vi "AlliGator Correct Dead Left Columns.vi"(8 "error in (no error)":errorcluster, 11 "Image Pixels":sgl[][](array[numeric])) -> (0 "error out":errorcluster, 3 "Corrected Image Pixels":sgl[][](array[numeric]))   [LabVIEW 2021, in "AlliGator Files.lvlib"]
doc: "Corrects for 1-every-other dead columns in the left half of a SPAD512S detector."
uses:
  AlliGator Files.lvlib
  35e40605-0482-421d-9502-94a1263c656b.vi
  <vilib>/Analysis/Matrix/Numeric/Conversions/Array To Matrix - RA2.vi
  <vilib>/Analysis/Matrix/Numeric/Conversions/Matrix To Array - RM.vi
  <vilib>/Analysis/Matrix/NI_Matrix.lvlib
panel:
  # "see the AlliGator License on the block diagram (Ctrl+E or Window:Show Block Diagram)"
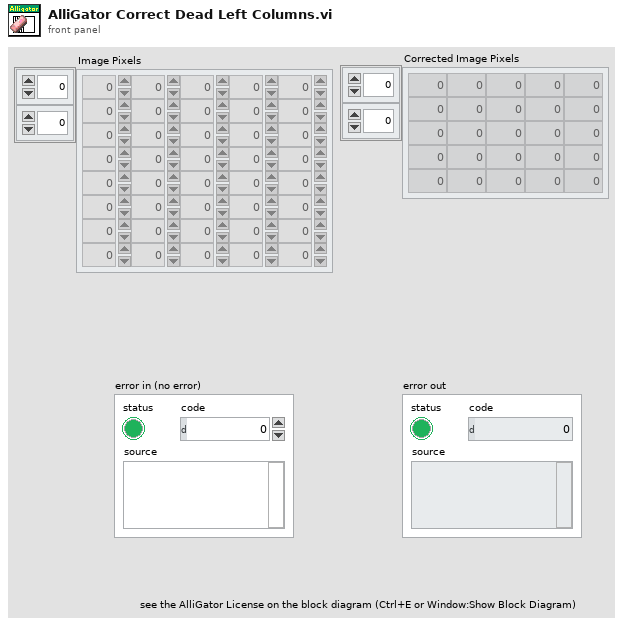
[diagram p1: front panel]
types:
  T1 = typedef "NI_Matrix.lvlib/RealMatrix.ctl" = dbl[][]
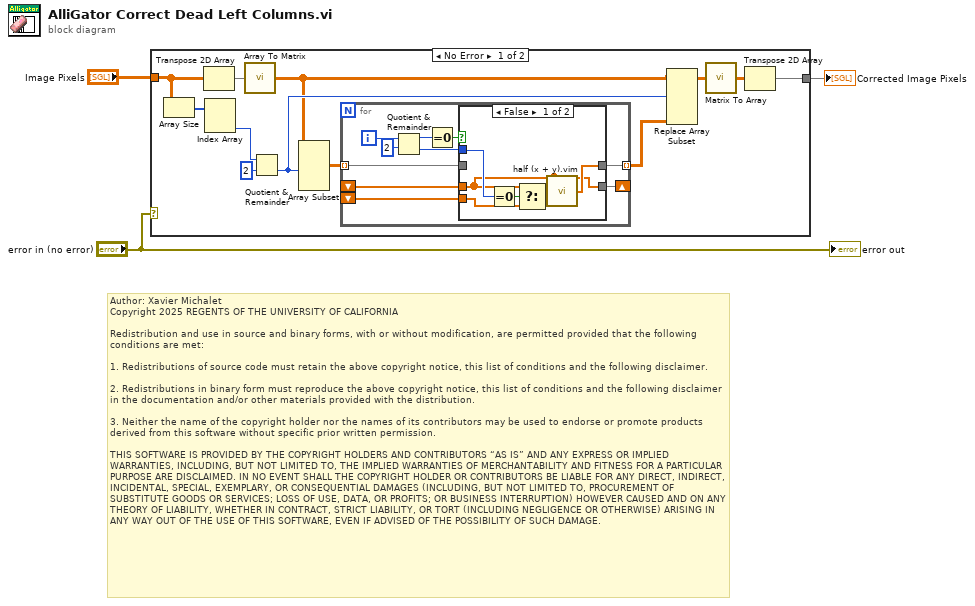
[diagram p0: block diagram]
diagram:
  # "Author: Xavier Michalet\nCopyright 2025 REGENTS OF THE UNIVERSITY OF CALIFORNIA\n\nRedistribution and use in source and binary forms, with or without modification, are permitted provided that the following conditions are met:\n\n1. Redistributions of source code must retain the above copyright notice, this list of conditions and the following disclaimer.\n\n2. Redistributions in binary form must reproduce the above copyright notice, this list of conditions and the following disclaimer in the documentation and/or other materials provided with the distribution.\n\n3. Neither the name of the copyright holder nor the names of its contributors may be used to endorse or promote products derived from this software without specific prior written permission.\n\nTHIS SOFTWARE IS PROVIDED BY THE COPYRIGHT HOLDERS AND CONTRIBUTORS “AS IS” AND ANY EXPRESS OR IMPLIED WARRANTIES, INCLUDING, BUT NOT LIMITED TO, THE IMPLIED WARRANTIES OF MERCHANTABILITY AND FITNESS FOR A PARTICULAR PURPOSE ARE DISCLAIMED. IN NO EVENT SHALL THE COPYRIGHT HOLDER OR CONTRIBUTORS BE LIABLE FOR ANY DIRECT, INDIRECT, INCIDENTAL, SPECIAL, EXEMPLARY, OR CONSEQUENTIAL DAMAGES (INCLUDING, BUT NOT LIMITED TO, PROCUREMENT OF SUBSTITUTE GOODS OR SERVICES; LOSS OF USE, DATA, OR PROFITS; OR BUSINESS INTERRUPTION) HOWEVER CAUSED AND ON ANY THEORY OF LIABILITY, WHETHER IN CONTRACT, STRICT LIABILITY, OR TORT (INCLUDING NEGLIGENCE OR OTHERWISE) ARISING IN ANY WAY OUT OF THE USE OF THIS SOFTWARE, EVEN IF ADVISED OF THE POSSIBILITY OF SUCH DAMAGE."
  n1 = case shown="No Error" "error in (no error)" {
    tunnel: "Image Pixels" -> [w13 w33]
    tunnel: [w8 w33] -> w2
    frame No Error {
      n2 = Array Size(array=w13) -> (size(s)=w15:i32[])
      n3 = Transpose 2D Array(2D array=w13) -> (transposed array=w10:sgl[][])
      n4 = Index Array(array=w15) -> (element #2=w9:i32)  [unwired: 2 in, 1 out]
      n5 = call-poly <vilib>:"Array To Matrix.vi"("Real 2D Array"=w10) -> ("Real Matrix"=w5:T1)
      n6 = Quotient & Remainder(x=w9, y=2) -> (floor(x/y)=w11:i32)  [unwired: 1 out]
      n7 = Array Subset(array=w5, length (row)=w11) -> (w7:T1)  [unwired: 3 in]
      n8 = for {
        tunnel: w7 -> [w22] mode=indexing
        tunnel: [w20] -> w6 mode=indexing
        shift-right: [w21] -> _
        shift-left: _ -> [w19]
        shift-left: _ -> [w18]
        i -> [w17]
        n9 = Quotient & Remainder(x=w17, y=2) -> (x-y*floor(x/y)=w24:i32, floor(x/y)=w16:i32)
        n10 = Equal To 0?(x=w24) -> (x = 0?=w23:bool)
        n11 = case shown="False" w23 {
          tunnel: w22 -> [_ w32]
          tunnel: [w26 w32] -> w21
          tunnel: [w28 w32] -> w20
          tunnel: w19 -> [w27 _]
          tunnel: w18 -> [w26 _]
          tunnel: w16 -> [w31 _]
          frame False {
            n12 = Equal To 0?(x=w31) -> (x = 0?=w30:bool)
            n13 = Select(t=w26, s=w30, f=w27) -> (s? t:f=w29:dbl[])
            n14 = call "half (x + y).vim"("y"=w29, "x"=w26) -> ("(x+y)/2"=w28:dbl[])  [unwired: 4 in]
          }
          frame True {
          }
        }
      }
      n15 = Replace Array Subset(array=w5, new element=w6, index (dim 1)=w11) -> (w12:T1)  [unwired: 3 in]
      n16 = call-poly <vilib>:"Matrix To Array.vi"("Real Matrix"=w12) -> ("Real 2D Array"=w4:dbl[][])
      n17 = Transpose 2D Array(2D array=w4) -> (transposed array=w8:dbl[][])
    }
    frame Error {
    }
  }
  "Corrected Image Pixels" <- w2
  "error out" <- "error in (no error)"
